vi "OpenRelay.vi"(8 "error in (no error)":errorcluster, 11 "device_info":cluster{}) -> (0 "error out":errorcluster, 2 "function return":i32, 3 "device_info out":cluster{})   [LabVIEW 2022 SP3, in "usb_relay_device.lvlib"]
doc: "int EXPORT_API usb_relay_device_open(struct usb_relay_device_info* device_info);"
uses:
  usb_relay_device.lvlib
  AppBuilderFiles/RunTimeExe/data/usb_relay_device.dll
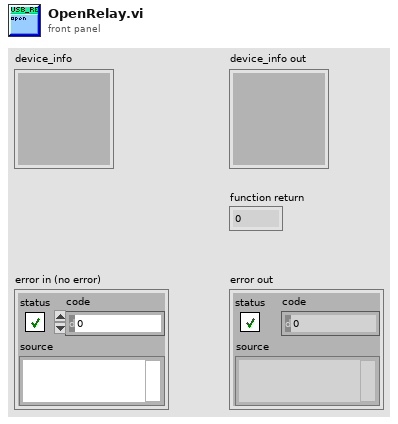
[diagram p1: front panel]
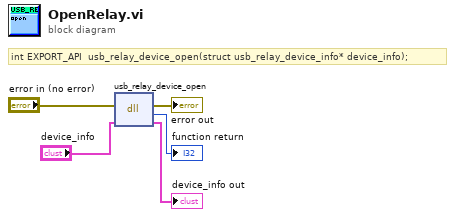
[diagram p0: block diagram]
diagram:
  # "int EXPORT_API  usb_relay_device_open(struct usb_relay_device_info* device_info);"
  n1 = dll-call lib="D:/LabVIEWSuite_64_OS/AppBuilderFiles/RunTimeExe/data/usb_relay_device.*" fn="usb_relay_device_open"(error in="error in (no error)", "device_info"="device_info") -> (error out=→"error out":errorcluster, →"function return":i32, "device_info"=→"device_info out":cluster{})  [unwired: 2 in, 1 out]
